vi "Get Actual Samp Rates Chassis.vi"(8 "error in (no error)":errorcluster, 10 "Chassis Cfg":refnum<class "ChassisCfg.lvclass">, 11 "Chassis Tasks in":refnum<class "Chassis Tasks.lvclass">) -> (0 "error out":errorcluster, 2 "Chassis Cfg":refnum<class "ChassisCfg.lvclass">, 3 "Chassis Tasks out":refnum<class "Chassis Tasks.lvclass">)   [LabVIEW 2018, in "Data Acquisition.lvlib" / "Chassis Tasks.lvclass"]
uses:
  Chassis Tasks.lvclass
  Cfg Grandmaster/Class Chassis Cfg/ChassisCfg.lvclass
  Chassis Tasks.lvclass/Chassis Tasks.ctl
  Common/Controls/TE_Designator.ctl
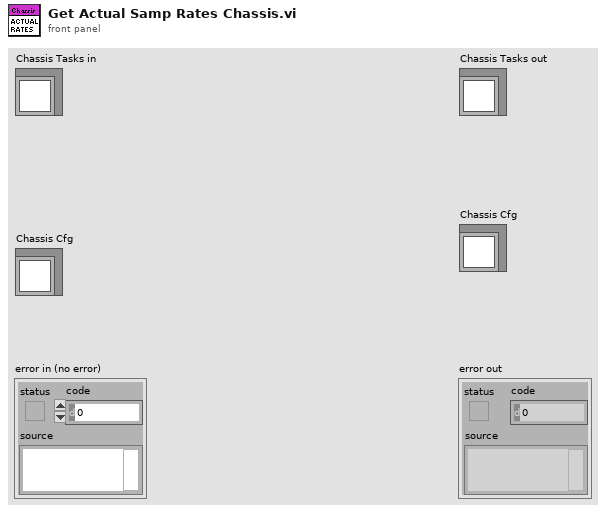
[diagram p1: front panel]
types:
  T1 = typedef "TE_Designator.ctl" = enum16{"High Speed", "Low Speed"}
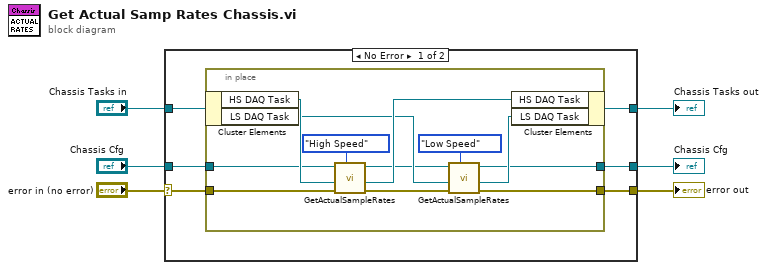
[diagram p0: block diagram]
diagram:
  n1 = case shown="No Error" "error in (no error)" {
    selector: "error in (no error)" -> [w11 w27]
    tunnel: [w10 w27] -> w5
    tunnel: [w8 w26] -> w3
    tunnel: "Chassis Tasks in" -> [w12 w26]
    tunnel: "Chassis Cfg" -> [w9 w25]
    tunnel: [w7 w25] -> w1
    frame No Error {
      n2 = in-place {
        in-place-border: w11 -> [w20]
        in-place-border: [w18] -> w10
        in-place-border: w9 -> [w17]
        in-place-border: [w15] -> w7
        n3 = in-place-cluster #1(w12) -> ("HS DAQ Task"=w24:refnum<class "DAQ Task.lvclass">, "LS DAQ Task"=w22:refnum<class "DAQ Task.lvclass">)
        n4 = call "GetActualSampleRates.vi"("TimingEngine"=TE_Designator."High Speed", "error in"=w20, "DAQ Task"=w24, "Chassis Cfg"=w17) -> ("error out"=w19:errorcluster, "DAQ Task"=w23:refnum<class "DAQ Task.lvclass">, "Chassis Cfg"=w16:refnum<class "ChassisCfg.lvclass">)  [unwired: 5 in]
        n5 = call "GetActualSampleRates.vi"("TimingEngine"=TE_Designator."Low Speed", "error in"=w19, "DAQ Task"=w22, "Chassis Cfg"=w16) -> ("error out"=w18:errorcluster, "DAQ Task"=w21:refnum<class "DAQ Task.lvclass">, "Chassis Cfg"=w15:refnum<class "ChassisCfg.lvclass">)  [unwired: 5 in]
        n6 = in-place-cluster #1("HS DAQ Task"=w23, "LS DAQ Task"=w21) -> (w8:refnum<class "Chassis Tasks.lvclass">)
      }
    }
    frame Error {
    }
  }
  "error out" <- w5
  "Chassis Tasks out" <- w3
  "Chassis Cfg" <- w1
